vi "MyTest_noeudCUDA.vi"(7 "CUDA Context out":refnum<class "CUDA Context.lvclass">, 8 "error IN":errorcluster, 11 "CDB *":T1 format="0x%016x") -> ()   [LabVIEW 2018]
uses:
  <vilib>/addons/lvgpu/lvcuda/CUDA Context/CUDA Context.lvclass
  <vilib>/addons/lvgpu/lvcuda/CUDA Device Ptr (CUdeviceptr).ctl
  <vilib>/addons/lvgpu/lvcuda/CUDA Context/Set Current Context (cuCtxSetCurrent).vi
  <vilib>/addons/lvgpu/lvcuda/Get Library Path.vi
  <vilib>/addons/lvgpu/lvcuda/Get Library Path - cuda.vi
  <vilib>/addons/lvgpu/lvcuda/CUDA Context/Get CUDA Context Properties.vi
  <vilib>/addons/lvgpu/lvcuda/NVIDIA CUDA Library Paths.vi
  <vilib>/addons/lvgpu/lvcuda/Convert Error Code.vi
  <vilib>/addons/lvgpu/lvcuda/Convert Error Code - cuda.vi
  <vilib>/addons/lvgpu/lvcuda.lvlib
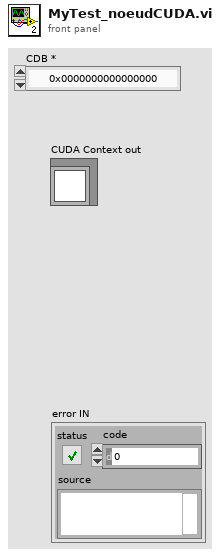
[diagram p1: front panel]
types:
  T1 = typedef "lvcuda.lvlib/CUDA Device Ptr (CUdeviceptr).ctl" = u64
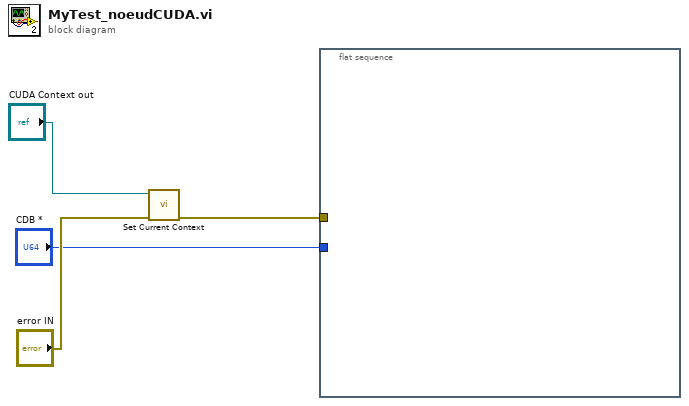
[diagram p0: block diagram]
diagram:
  n1 = call <vilib>:"Set Current Context.vi"("error in"="error IN", "CUDA Context in"="CUDA Context out") -> ("error out"=w1:errorcluster)  [unwired: 7 in, 2 out]
  n2 = flat-sequence {
    tunnel: "CDB *" -> [_]
    tunnel: w1 -> [_]
    frame #0 {
    }
  }
